vi "user initialization.vi"(8 "error in":errorcluster, 10 "configuration in":refnum<class "control module configuration.lvclass">, 11 "fixed channel runtime in":refnum<class "WaveformAcq runtime.lvclass">) -> (0 "error out":errorcluster, 3 "fixed channel runtime out":refnum<class "WaveformAcq runtime.lvclass">)   [LabVIEW 2017, in "WaveformAcq runtime.lvclass"]
uses:
  WaveformAcq runtime.lvclass
  <vilib>/NI/DCAF/Tag Editor Core/control module/configuration/control module configuration.lvclass
  <vilib>/userdefined/High Color/nirio_resource_hc.ctl
  <vilib>/NI/DCAF/addons/InstructionFrameworkSupport/FPGA_FGV_action.ctl
  configuration/WaveformAcq configuration.lvclass
  C:/Program Files (x86)/National Instruments/LabVIEW 2017/vi.lib/NI/DCAF/Tag Editor Core/control module/configuration/control module configuration.lvclass
  configuration/WaveformAcq configuration.lvclass/WaveformAcq configuration.ctl
  WaveformAcq runtime.lvclass/WaveformAcq runtime.ctl
  <vilib>/NI/DCAF/Tag Editor Core/control module/runtime/control module runtime.lvclass
  <vilib>/NI/PowerElectronicsControl/WaveformAcq/RT/WaveformTask.lvclass
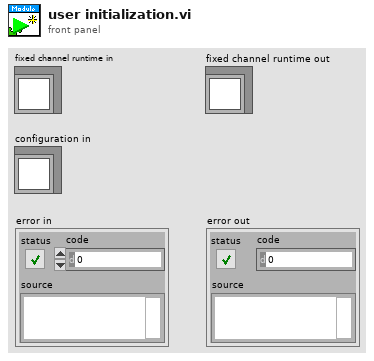
[diagram p1: front panel]
types:
  T1 = typedef "FPGA_FGV_action.ctl" = enum16{"get FPGA", "set FPGA", "Close"}
  T2 = typedef "nirio_resource_hc.ctl" = tag
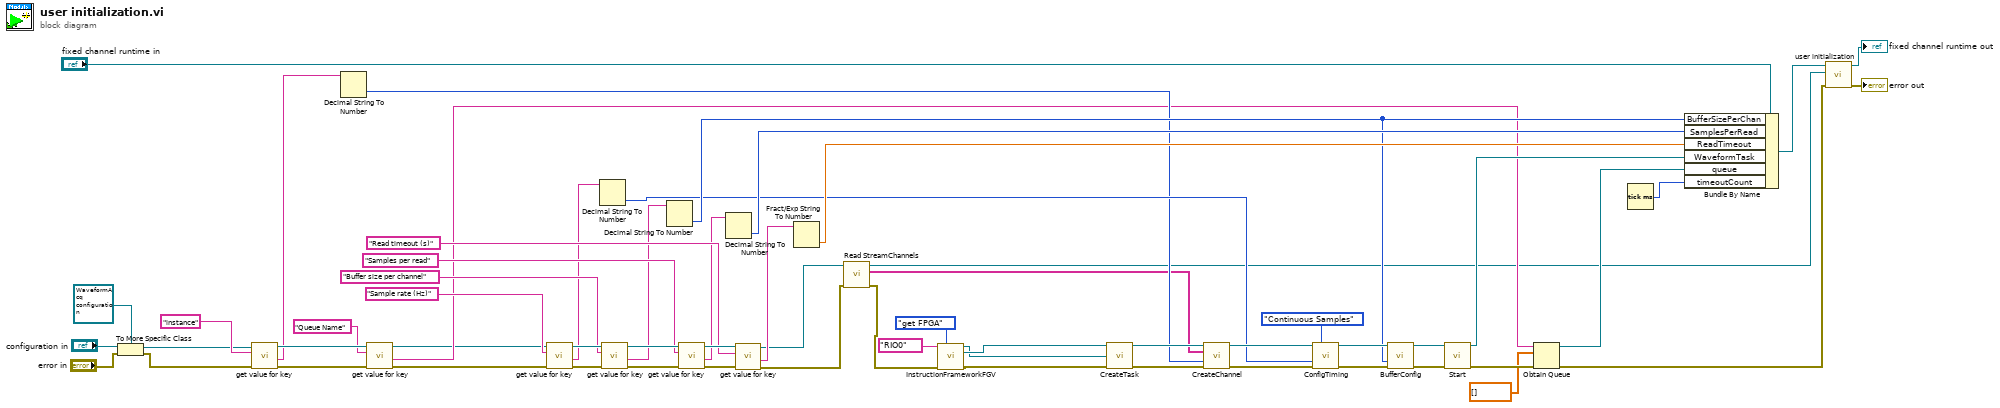
[diagram p0: block diagram]
diagram:
  n1 = To More Specific Class(target class=refnum<class "WaveformAcq configuration.lvclass"> refnum ("WaveformAcq configuration"), reference="configuration in", error in="error in") -> (specific class reference=w8:refnum<class "WaveformAcq configuration.lvclass">, error out=w6:errorcluster)
  n2 = call-dynamic "get value for key.vi"("error in"=w6, "key"="instance", "fixed channel configuration in"=w8) -> ("error out"=w57:errorcluster, "value"=w36:string, "fixed channel configuration out"=w58:refnum<class "WaveformAcq configuration.lvclass">)  [unwired: 6 in]
  n3 = Decimal String To Number(string=w36) -> (number=w24:i32)  [unwired: 2 in, 1 out]
  n4 = call-dynamic "get value for key.vi"("error in"=w57, "key"="Queue Name" ("String"), "fixed channel configuration in"=w58) -> ("error out"=w12:errorcluster, "value"=w21:string, "fixed channel configuration out"=w11:refnum<class "WaveformAcq configuration.lvclass">)  [unwired: 6 in]
  n5 = call-dynamic "get value for key.vi"("error in"=w12, "key"="Sample rate (Hz)" ("String"), "fixed channel configuration in"=w11) -> ("error out"=w53:errorcluster, "value"=w33:string, "fixed channel configuration out"=w55:refnum<class "WaveformAcq configuration.lvclass">)  [unwired: 6 in]
  n6 = Decimal String To Number(string=w33) -> (number=w26:i32)  [unwired: 2 in, 1 out]
  n7 = call-dynamic "get value for key.vi"("error in"=w53, "key"="Buffer size per channel" ("String"), "fixed channel configuration in"=w55) -> ("error out"=w52:errorcluster, "value"=w32:string, "fixed channel configuration out"=w54:refnum<class "WaveformAcq configuration.lvclass">)  [unwired: 6 in]
  n8 = Decimal String To Number(string=w32) -> (number=w27:i32)  [unwired: 2 in, 1 out]
  n9 = call-dynamic "get value for key.vi"("error in"=w52, "key"="Samples per read" ("String"), "fixed channel configuration in"=w54) -> ("error out"=w47:errorcluster, "value"=w31:string, "fixed channel configuration out"=w48:refnum<class "WaveformAcq configuration.lvclass">)  [unwired: 6 in]
  n10 = Decimal String To Number(string=w31) -> (number=w29:i32)  [unwired: 2 in, 1 out]
  n11 = call-dynamic "get value for key.vi"("error in"=w47, "key"="Read timeout (s)" ("String"), "fixed channel configuration in"=w48) -> ("error out"=w2:errorcluster, "value"=w30:string, "fixed channel configuration out"=w5:refnum<class "WaveformAcq configuration.lvclass">)  [unwired: 6 in]
  n12 = Fract/Exp String To Number(string=w30) -> (number=w28:dbl)  [unwired: 3 in, 1 out]
  n13 = call "Read StreamChannels.vi"("error in (no error)"=w2, "WaveformAcq configuration in"=w5) -> ("error out"=w1:errorcluster, "StreamChannels"=w4:string[], "WaveformAcq configuration out"=w3:refnum<class "WaveformAcq configuration.lvclass">)  [unwired: 7 in]
  n14 = call <vilib>:"InstructionFrameworkFGV.vi"("RIO resource"=T2 "RIO0", "Action"=FPGA_FGV_action."get FPGA", "error in"=w1) -> ("session out"=w14:refnum<class "niInstr FIFO Register Bus v1 Host.lvclass">, "bitfile"=w15:refnum<k20>, "error out"=w16:errorcluster)  [unwired: 10 in]
  n15 = call <vilib>:"CreateTask.vi"("FPGA Ref in"=w15, "session in"=w14, "error in"=w16) -> ("Task out"=w38:refnum<class "WaveformTask.lvclass">, "error out"=w37:errorcluster)  [unwired: 9 in, 2 out]
  n16 = call <vilib>:"CreateChannel.vi"("task in"=w38, "Chan Name Array"=w4, "instance"=w24, "error in"=w37) -> ("Task out"=w39:refnum<class "WaveformTask.lvclass">, "error out"=w45:errorcluster)  [unwired: 10 in]
  n17 = call <vilib>:"ConfigTiming.vi"("Task in"=w39, "Sample Mode"=enum16{"Finite Samples", "Continuous Samples"}."Continuous Samples", "Sample Rate"=w26, "error in (no error)"=w45) -> ("Task out"=w43:refnum<class "WaveformTask.lvclass">, "error out"=w42:errorcluster)  [unwired: 9 in, 1 out]
  n18 = call <vilib>:"BufferConfig.vi"("WaveformTask in"=w43, "Buffer Size [Samps per Chan]"=w27, "error in (no error)"=w42) -> ("WaveformTask out"=w41:refnum<class "WaveformTask.lvclass">, "error out"=w40:errorcluster)  [unwired: 10 in, 1 out]
  n19 = call <vilib>:"Start.vi"("WaveformTask in"=w41, "error in (no error)"=w40) -> ("WaveformTask out"=w25:refnum<class "WaveformTask.lvclass">, "error out"=w23:errorcluster)  [unwired: 12 in]
  n20 = Obtain Queue(name (unnamed)=w21, element data type=sgl[] [], error in (no error)=w23) -> (queue out=w19:refnum<queue>, error out=w22:errorcluster)  [unwired: 2 in, 1 out]
  n21 = Tick Count (ms)() -> (millisecond timer value=w13:u32)
  n22 = Bundle By Name(cluster="fixed channel runtime in", "BufferSizePerChan"=w27, "SamplesPerRead"=w29, "ReadTimeout"=w28, "WaveformTask"=w25, "queue"=w19, "timeoutCount"=w13) -> (w34:refnum<class "WaveformAcq runtime.lvclass">)
  n23 = call-parent "user initialization.vi"("error in"=w22, "configuration in"=w3, "fixed channel runtime in"=w34) -> ("error out"=→"error out":errorcluster, "fixed channel runtime out"=→"fixed channel runtime out":refnum<class "WaveformAcq runtime.lvclass">)  [unwired: 7 in]
